vi "MuxSwitchSingle.vi"(7 "MUX address":u32=1 min=1 max=12 step=1, 8 "error in (no error)":errorcluster, 9 "Channel":i32=1 min=1 max=12 step=1, 10 "C1 / C2":i32=1 min=1 max=12 step=1, 11 "Pickering in":refnum<class "Pickering.lvclass">) -> (0 "error out":errorcluster, 2 "command string":string, 3 "Pickering out":refnum<class "Pickering.lvclass">)   [LabVIEW 2019, in "Pickering.lvclass"]
uses:
  Pickering.lvclass
  C:/Users/probe/Desktop/TRIUMF-Dark-Box/InstrControl/InstrControl.lvclass
  PickeringMUX_CommandsGlobal.vi
  InstrControl.lvclass
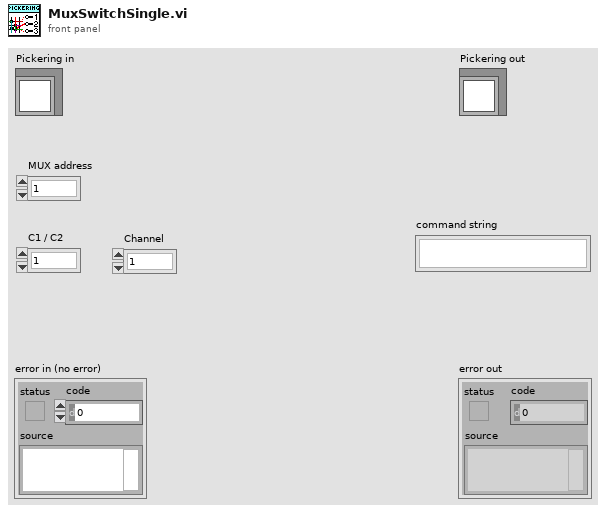
[diagram p1: front panel]
types:
  T1 = cluster{"Mux1 address":string, "Mux2 address":string, "Instrument name":string, "Instrument type":u16, "Command \"MUX Reset\"":string, "Command \"Select MUX Channel\"":string}
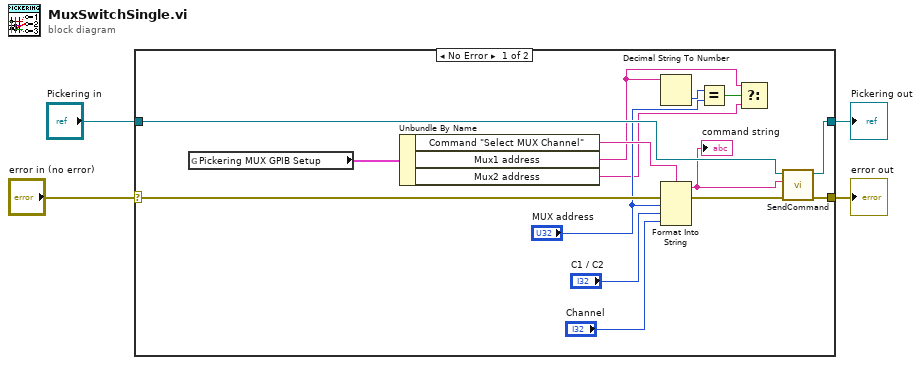
[diagram p0: block diagram]
diagram:
  n1 = case shown="No Error" "error in (no error)" {
    selector: "error in (no error)" -> [w18 w21]
    tunnel: "Pickering in" -> [w16 w20]
    tunnel: [w15 w21] -> w2
    tunnel: [w14 w20] -> w1
    frame No Error {
      n2 = global read "PickeringMUX_CommandsGlobal.vi" "Pickering MUX GPIB Setup"() -> (w19:T1)
      n3 = Unbundle By Name(w19) -> ("Command \"Select MUX Channel\""=w11:string, "Mux1 address"=w6:string, "Mux2 address"=w7:string)
      n4 = Decimal String To Number(string=w6) -> (number=w10:i32)  [unwired: 2 in, 1 out]
      n5 = Format Into String(format string=w11, error in=w18, "MUX address", "C1 / C2", "Channel") -> (resulting string=w5:string, error out=w17:errorcluster)  [unwired: 1 in]
      "command string" <- w5
      n6 = Equal?(x=w10, y="MUX address") -> (x = y?=w8:bool)
      n7 = Select(t=w6, s=w8, f=w7) -> ()  [unwired: 1 out]
      n8 = call "SendCommand.vi"("error in (no error)"=w17, "Command string"=w5, "InstControl in"=w16) -> ("error out"=w15:errorcluster, "InstControl out"=w14:refnum<class "Pickering.lvclass">)  [unwired: 7 in]
    }
    frame Error {
    }
  }
  "error out" <- w2
  "Pickering out" <- w1
